vi "WriteCount.vi"(8 "error in (no error)":errorcluster, 10 "Count":i32, 11 "DisplayUI in":refnum<class "DisplayUI.lvclass">) -> (0 "error out":errorcluster, 3 "DisplayUI out":refnum<class "DisplayUI.lvclass">)   [LabVIEW 2013, in "DisplayUI.lvclass"]
uses:
  DisplayUI.lvclass
  DisplayUI.lvclass/DisplayUI.ctl
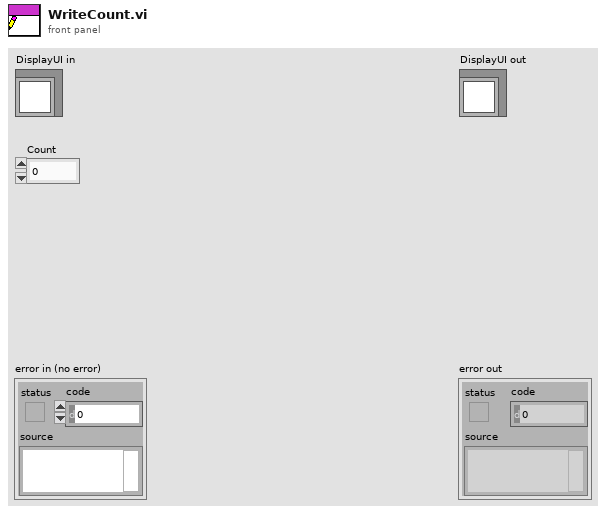
[diagram p1: front panel]
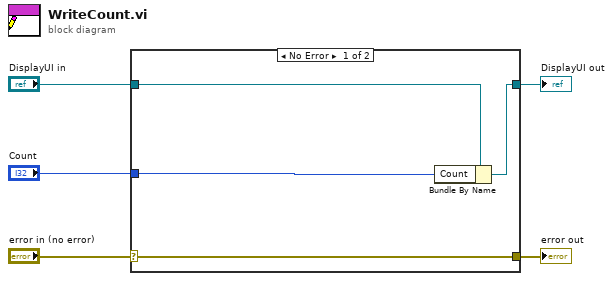
[diagram p0: block diagram]
diagram:
  n1 = case shown="No Error" "error in (no error)" {
    selector: "error in (no error)" -> [w9 w10]
    tunnel: [w9 w10] -> w4
    tunnel: [w7 w11] -> w2
    tunnel: "DisplayUI in" -> [w8 w11]
    tunnel: "Count" -> [w6 _]
    frame No Error {
      n2 = Bundle By Name(cluster=w8, "Count"=w6) -> (w7:refnum<class "DisplayUI.lvclass">)
    }
    frame Error {
    }
  }
  "error out" <- w4
  "DisplayUI out" <- w2
